vi "FlatToRichni_measurementlink_sessionmanagement_v1_ReserveAllRegisteredSessionsResponse.vi"(5 "OutputClusterType":T1, 11 "InputCluster":T5) -> (3 "OutputCluster":T1)   [LabVIEW 2020, in "ni.measurementlink.sessionmanagement.v1.lvlib"]
uses:
  ni.measurementlink.sessionmanagement.v1.lvlib
  ni_measurementlink_sessionmanagement_v1_ReserveAllRegisteredSessionsResponse_Flat.ctl
  ni_measurementlink_sessionmanagement_v1_SessionInformation_Flat.ctl
  nidevice_grpc_Session_Flat.ctl
  ni_measurementlink_sessionmanagement_v1_ChannelMapping_Flat.ctl
  ni_measurementlink_sessionmanagement_v1_ReserveAllRegisteredSessionsResponse.ctl
  ni_measurementlink_sessionmanagement_v1_SessionInformation.ctl
  nidevice_grpc_Session.ctl
  ni_measurementlink_sessionmanagement_v1_ChannelMapping.ctl
  FlatToRichnidevice_grpc_Session.vi
  FlatToRichni_measurementlink_sessionmanagement_v1_ChannelMapping.vi
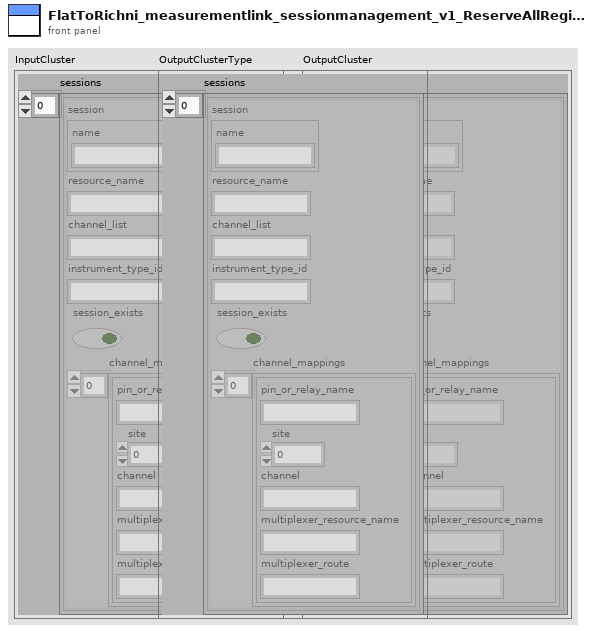
[diagram p1: front panel]
types:
  T1 = typedef "ni.measurementlink.sessionmanagement.v1.lvlib/ni_measurementlink_sessionmanagement_v1_ReserveAllRegisteredSessionsResponse.ctl" = cluster{"sessions":T2[]}
  T2 = typedef "ni.measurementlink.sessionmanagement.v1.lvlib/ni_measurementlink_sessionmanagement_v1_SessionInformation.ctl" = cluster{"session":T3, "resource_name":string, "channel_list":string, "instrument_type_id":string, "session_exists":bool, "channel_mappings":T4[]}
  T3 = typedef "ni.measurementlink.sessionmanagement.v1.lvlib/nidevice_grpc_Session.ctl" = cluster{"name":string}
  T4 = typedef "ni.measurementlink.sessionmanagement.v1.lvlib/ni_measurementlink_sessionmanagement_v1_ChannelMapping.ctl" = cluster{"pin_or_relay_name":string, "site":i32, "channel":string, "multiplexer_resource_name":string, "multiplexer_route":string}
  T5 = typedef "ni.measurementlink.sessionmanagement.v1.lvlib/ni_measurementlink_sessionmanagement_v1_ReserveAllRegisteredSessionsResponse_Flat.ctl" = cluster{"sessions":T6[]}
  T6 = typedef "ni.measurementlink.sessionmanagement.v1.lvlib/ni_measurementlink_sessionmanagement_v1_SessionInformation_Flat.ctl" = cluster{"session":T7, "resource_name":string, "channel_list":string, "instrument_type_id":string, "session_exists":bool, "channel_mappings":T8[]}
  T7 = typedef "ni.measurementlink.sessionmanagement.v1.lvlib/nidevice_grpc_Session_Flat.ctl" = cluster{"name":string}
  T8 = typedef "ni.measurementlink.sessionmanagement.v1.lvlib/ni_measurementlink_sessionmanagement_v1_ChannelMapping_Flat.ctl" = cluster{"pin_or_relay_name":string, "site":i32, "channel":string, "multiplexer_resource_name":string, "multiplexer_route":string}
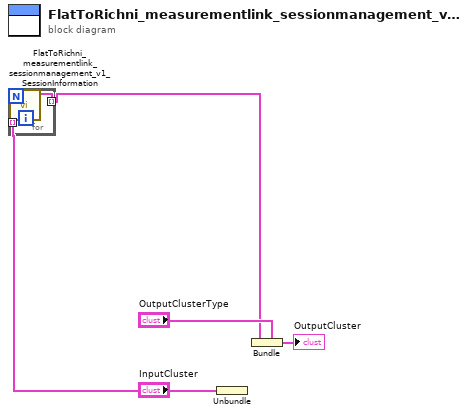
[diagram p0: block diagram]
diagram:
  n1 = Unbundle "Unbundle"("InputCluster") -> ("sessions"=w2:T6[])
  n2 = for {
    tunnel: w2 -> [w7] mode=indexing
    tunnel: [w6] -> w1 mode=indexing
    n3 = call "FlatToRichni_measurementlink_sessionmanagement_v1_SessionInformation.vi"("InputCluster"=w7) -> ("OutputCluster"=w6:T2)  [unwired: 10 in]
  }
  n4 = Bundle "Bundle"(cluster="OutputClusterType", "sessions"=w1) -> (→"OutputCluster":T1)
